vi "Index finden.vi"() -> (3 "Index":i32)   [LabVIEW 2020, in "Regler.lvlib" / "Druckregler.lvlib"]
uses:
  Druckregler.lvlib
  Allgemein/FGV Zustaende Aktionen.ctl
  Konfig-Dateien/FGV Betriebsdaten Aktionen.ctl
  Allgemein/Allgemein.lvlib
  Konfig-Dateien/Konfig-Dateien.lvlib
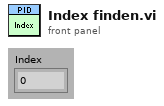
[diagram p1: front panel]
types:
  T1 = typedef "Konfig-Dateien.lvlib/FGV Betriebsdaten Aktionen.ctl" = enum16{"lesen", "Anlagengrenzw.", "PID Param.", "Sonstige", "Sensor Para."}
  T2 = typedef "Allgemein.lvlib/FGV Zustaende Aktionen.ctl" = enum16{"lesen", "Zustand PC", "Zustand cRIO", "Bildnummer", "Samplepoint", "Sysloglevel"}
  T3 = typedef "Anlagengrenzwerte.lvlib/Anlagen-Grenzwerte Anzeige.ctl" = cluster{"Eingangsdruck FT-IR:":T4, "Durchfluss FT-IR:":T4, "Durchfluss CalGas:":T4, "Druck Ausgang:":T4, "Druck Kalter Block:":T4, "Heizleitungen intern:":T4, "Heizleitung zu FT-IR:":T4, "Heizung Filterblock:":T4, "Heizung Pumpe:":T4, "Heizleitung Extern SP1:":T4, "Heizleitung Extern SP2:":T4, "FT-IR Heizung Messzelle:":T4, "Schaltschranktemperatur:":T4, "Gaskühler:":T4}
  T4 = typedef "Anlagengrenzwerte.lvlib/Anlagen-Parameter Anzeige.ctl" = cluster{"Sollwert":sgl, "Warn-Min":sgl, "Warn-Max":sgl, "Abschalt-Min":sgl, "Abschalt-Max":sgl, "Regler":u16}
  T5 = typedef "Funktionstasten.lvlib/Zustaende.ctl" = enum16{"Standby", "Pause", "Eco", "Messen", "Kalibrieren", "Spülen Filter", "Spülen Leitung", "Umgebungsluft", "0-Gas", "Cal-Gas", "CG zu PNS", "-------------", "Init 1", "Init 2", "Init 3", "Init 4", "Messen vorbereiten", "Messen durchführen", "Exit"}
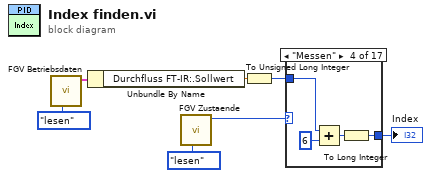
[diagram p0: block diagram]
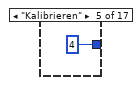
[diagram p5: hidden frame]
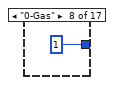
[diagram p8: hidden frame]
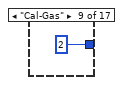
[diagram p9: hidden frame]
diagram:
  n1 = call "FGV Betriebsdaten.vi"("Aktionen"=FGV_Betriebsdaten_Aktionen."lesen") -> ("Anlagen-Grenzwerte"=w1:T3)  [unwired: 7 in, 3 out]
  n2 = Unbundle By Name(w1) -> ("Durchfluss FT-IR:.Sollwert"=w6:sgl)
  n3 = call "FGV Zustaende.vi"("Aktionen"=FGV_Zustaende_Aktionen."lesen") -> ("Zustand PC"=w3:T5)  [unwired: 6 in, 4 out]
  n4 = To Unsigned Long Integer(number=w6) -> (unsigned 32bit integer=w5:u32)
  n5 = case shown="\"Messen\"" w3 {
    tunnel: [_ _ _ w8 4 ("Index") _ _ 1 ("Index") 2 ("Index") _ _ _ _ _ _ _ _] -> w7
    tunnel: w5 -> [_ _ _ w11 _ _ _ _ _ _ _ _ _ _ _ _ _]
    frame "Standby", Default {
    }
    frame "Pause" {
    }
    frame "Eco" {
    }
    frame "Messen" {
      n6 = Add(x=w11, y=u32 6) -> (x+y=w9:u32)
      n7 = To Long Integer(number=w9) -> (32bit integer=w8:i32)
    }
    frame "Kalibrieren" {
    }
    frame "Spülen Filter" {
    }
    frame "Spülen Leitung" {
    }
    frame "0-Gas" {
    }
    frame "Cal-Gas" {
    }
    frame "-------------" {
    }
    frame "Init 1" {
    }
    frame "Init 2" {
    }
    frame "Init 3" {
    }
    frame "Init 4" {
    }
    frame "Messen vorbereiten" {
    }
    frame "Messen durchführen" {
    }
    frame "Exit" {
    }
  }
  "Index" <- w7
